vi "Initialize.vi"(8 "error in":errorcluster, 11 "Data Subject in":refnum<class "Data Subject.lvclass">) -> (0 "error out":errorcluster, 2 "DVR":refnum<data-value>, 3 "Data Subject out":refnum<class "Data Subject.lvclass">)   [LabVIEW 2015, in "Data Subject.lvclass"]
doc: "This VI must be overridden to provide useful feedback but the parent will provide a reference for a stop occurrence that can be used by the children. Children should provide a reference to the proper data object (loading it into the subject class). The specific data object must be downcasted to the generic data object."
uses:
  Data Subject.lvclass
  Data/Data.lvclass
  Data Subject.lvclass/Data Subject.ctl
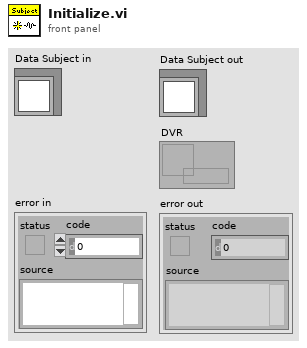
[diagram p1: front panel]
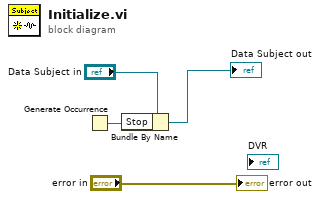
[diagram p0: block diagram]
diagram:
  n1 = Generate Occurrence() -> (w1:refnum<k4>)
  n2 = Bundle By Name(cluster="Data Subject in", "Stop"=w1) -> (→"Data Subject out":refnum<class "Data Subject.lvclass">)
  "error out" <- "error in"
